vi "Case Selection.vi"(8 "error in (no error)":errorcluster, 9 "Status_Cluster_in":T1={"simTime"=0.0, "simFrame"=0.0, "Connection Status"=enum."Disconnected", "Connection Command"=enum."Disconnect", "Last Error"=0, "Case selection"=enum."Connecting"}) -> (0 "error out":errorcluster, 1 "Status_Cluster_out":T1={"simTime"=0.0, "simFrame"=0.0, "Connection Status"=enum."Disconnected", "Connection Command"=enum."Disconnect", "Last Error"=0, "Case selection"=enum."Connecting"})   [LabVIEW 2020, in "Vires VTD Engine.lvlib"]
doc: "Reads the connection command + the connection status and the last error out of the status cluster and makes decision on the case selection for the next iteration"
uses:
  Vires VTD Engine.lvlib
  Type/Status_Cluster.ctl
  Type/ConnectionStatus.ctl
  Type/CaseSelection.ctl
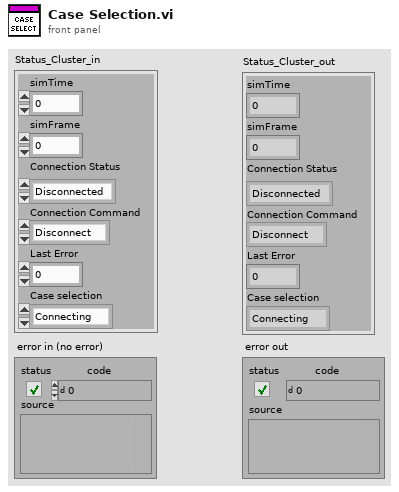
[diagram p1: front panel]
types:
  T1 = typedef "Vires VTD Engine.lvlib/Status_Cluster.ctl" = cluster{"simTime":dbl, "simFrame":dbl, "Connection Status":T2, "Connection Command":enum16{"Disconnect", "Connect"}, "Last Error":i32, "Case selection":T3}
  T2 = typedef "Vires VTD Engine.lvlib/ConnectionStatus.ctl" = enum16{"Disconnected", "Connected"}
  T3 = typedef "Vires VTD Engine.lvlib/CaseSelection.ctl" = enum32{"Idle", "Connecting", "Disconnecting", "Read/Write"}
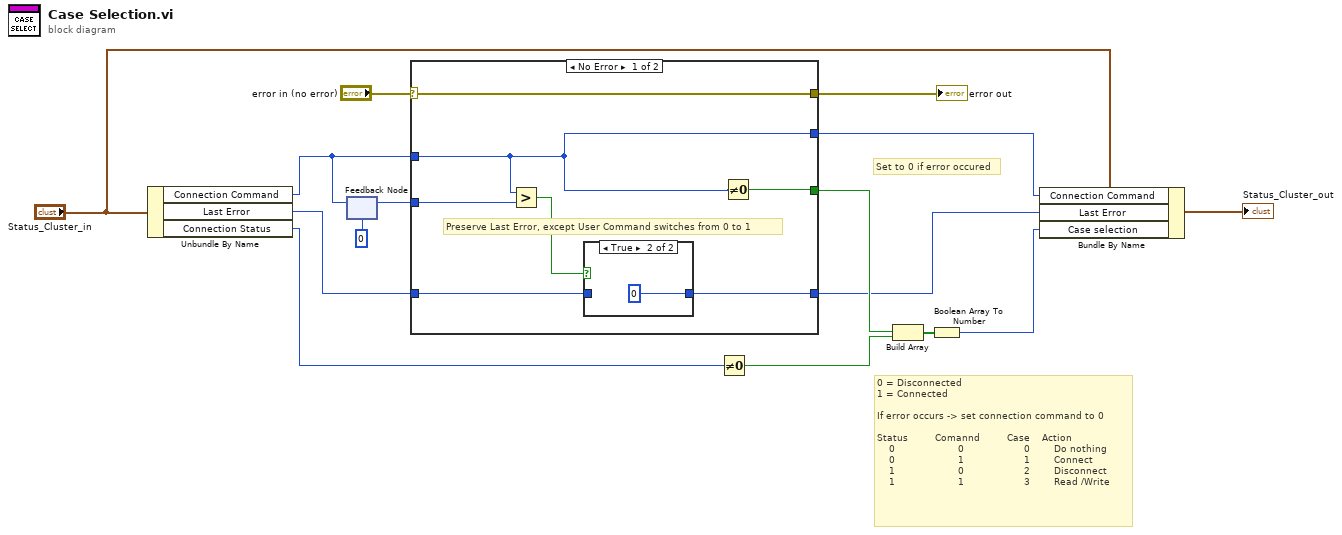
[diagram p0: block diagram]
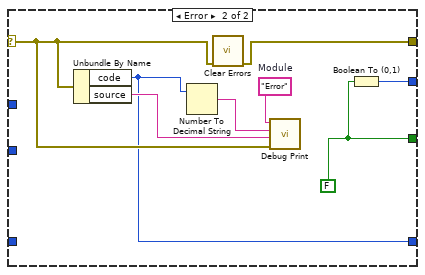
[diagram p3: hidden frame]
diagram:
  # "Set to 0 if error occured"
  # "0 = Disconnected\n1 = Connected\n\nIf error occurs -> set connection command to 0 \n\nStatus         Comannd         Case    Action\n    0                     0                    0        Do nothing\n    0                     1                    1        Connect\n    1                     0                    2        Disconnect\n    1                     1                    3        Read /Write"
  n1 = Unbundle By Name("Status_Cluster_in") -> ("Connection Command"=w8:enum16{"Disconnect", "Connect"}, "Last Error"=w7:i32, "Connection Status"=w6:T2)
  n2 = feedback #1(0) -> (w10:i32)
  n3 = feedback-in #1(w8) -> ()
  n4 = case shown="No Error" "error in (no error)" {
    selector: "error in (no error)" -> [w22 w31]
    tunnel: [w21 w26] -> w14
    tunnel: [w22 w32] -> w12
    tunnel: [w17 w29] -> w2
    tunnel: w8 -> [w20 _]
    tunnel: [w20 w27] -> w3
    tunnel: w7 -> [w18 _]
    tunnel: w10 -> [w16 _]
    frame No Error {
      # "Preserve Last Error, except User Command switches from 0 to 1"
      n5 = Greater?(x=w20, y=w16) -> (0:w19:bool)
      n6 = case shown="True" w19 {
        tunnel: w18 -> [w23 _]
        tunnel: [w23 0] -> w17
        frame False {
        }
        frame True {
        }
      }
      n7 = Not Equal To 0?(x=w20) -> (x != 0?=w21:bool)
    }
    frame Error {
      w25 = "Error"  # Module
      w26 = FALSE
      n8 = Unbundle By Name(w31) -> ("code"=w29:i32, "source"=w30:string)
      n9 = Number To Decimal String(number=w29) -> (decimal integer string=w28:string)  [unwired: 1 in]
      n10 = call <vilib>:"Clear Errors.vi"("error in (no error)"=w31) -> ("error out"=w32:errorcluster)  [unwired: 5 in, 1 out]
      n11 = call "Debug Print.vi"("error out"=w31, "comment"=w30, "Index"=w28, "Module"=w25) -> ()  [unwired: 8 in]
      n12 = Boolean To (0,1)(Boolean=w26) -> (0, 1=w27:i16)
    }
  }
  "error out" <- w12
  n13 = Not Equal To 0?(x=w6) -> (x != 0?=w11:bool)
  n14 = Build Array(w14, w11) -> (w15:bool[])
  n15 = Boolean Array To Number(Boolean array=w15) -> (number=w1:u32)
  n16 = Bundle By Name(cluster="Status_Cluster_in", "Connection Command"=w3, "Last Error"=w2, "Case selection"=w1) -> (→"Status_Cluster_out":T1)
